vi "Chart Main LV2012 NIVerified.vi"() -> ()   [LabVIEW 2016]
panel:
  in  "Open Graph Window":bool
  in  "stop":bool
  # "Overview: Sometimes, the subVI settings for Show Front Panel When Called/Run don't provide the flexibility or control you need for your application. In these cases you can use VI Server to control the window state.\nRequirements:\nLabVIEW 2012 (or compatible)\nInstructions:\nRun this VI"
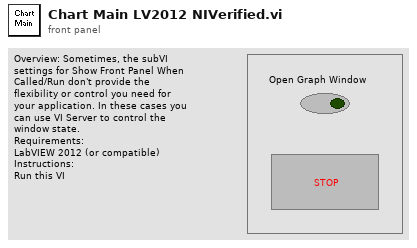
[diagram p1: front panel]
types:
  T1 = enum32{"Invalid", "Standard", "Closed", "Hidden", "Minimized", "Maximized"}
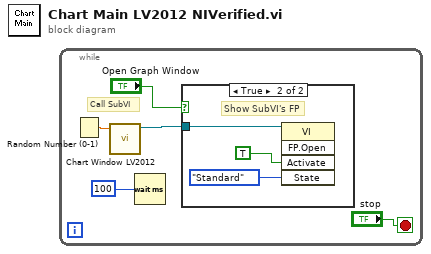
[diagram p0: block diagram]
diagram:
  n1 = while {
    stop <- "stop" stop-if-true
    # "Call SubVI"
    n2 = Random Number (0-1)() -> (number: 0 to 1=w4:dbl)
    n3 = call "Chart Window LV2012.vi"("Numeric"=w4) -> ("This VI"=w3:refnum<vi>)  [unwired: 10 out]
    n4 = Wait (ms)(milliseconds to wait=u32 100) -> ()  [unwired: 1 out]
    n5 = case shown="True" "Open Graph Window" {
      tunnel: w3 -> [_ w8]
      frame False {
      }
      frame True {
        # "Show SubVI's FP"
        n6 = invoke class="VI" method="FP.Open"(reference=w8, "Activate"=TRUE ("Activate?"), "State"=T1."Standard") -> ()  [unwired: 2 in, 5 out]
      }
    }
  }
